vi "OuputFormater.vi"(9 "Sine in":fxp<+/-,16,0>[](array[numeric])=[0.0, 0.0, 0.0, 0.0, 0.0, 0.0, 0.0, 0.0], 10 "Cosine in":fxp<+/-,16,0>[](array[numeric])=[0.0, 0.0, 0.0, 0.0, 0.0, 0.0, 0.0, 0.0]) -> (3 "test":i16[](array[numeric]))   [LabVIEW 2013]
doc: "Outputs input from channel 0 as I*cos(t)-Q*sin(t) on analog output 0"
uses:
  <vilib>/eio/EIONode/EIONode.xnode
  <vilib>/rvi/FXPMathLib/FxpInterpret/XNode/nifxpmath_Interpret.xnode
  <vilib>/rvi/eio/common/nirviEmuTemplateMethod_errors.vi
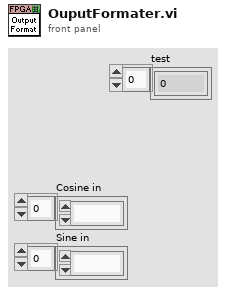
[diagram p1: front panel]
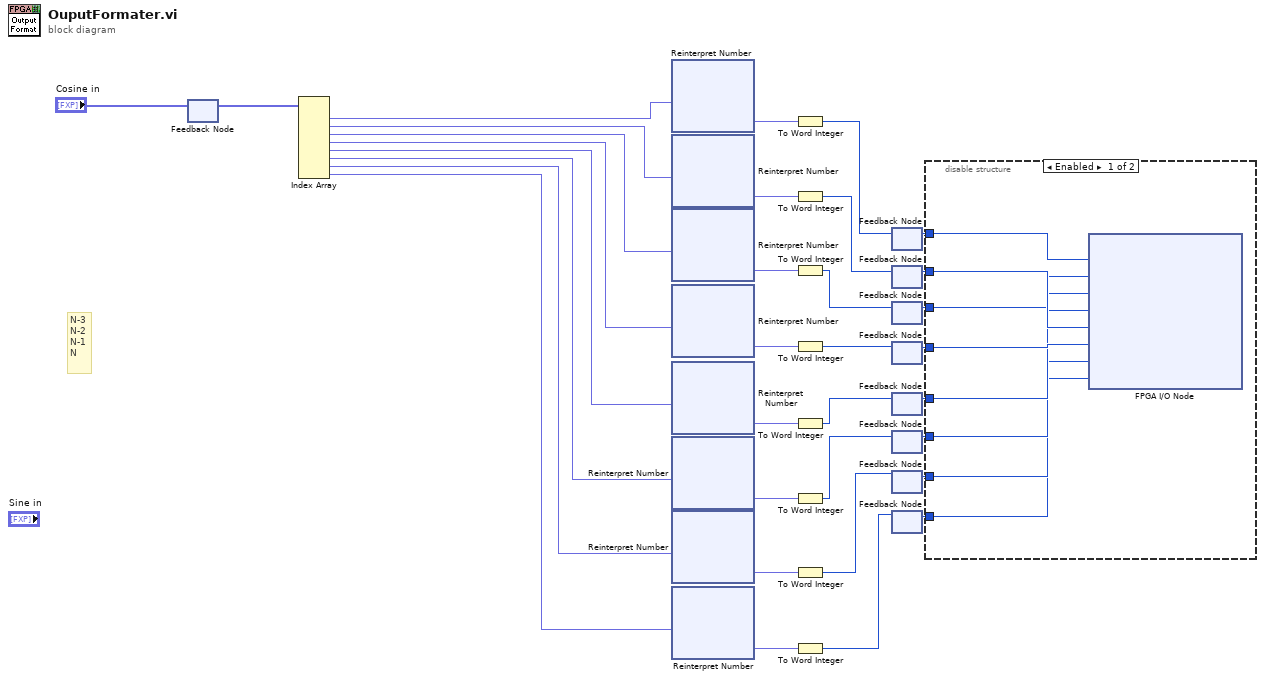
[diagram p0: block diagram]
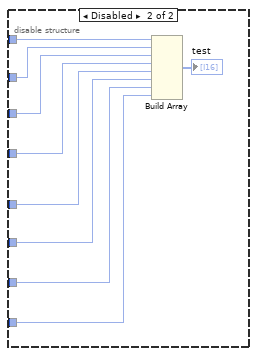
[diagram p2: hidden frame]
diagram:
  # "N-3\nN-2\nN-1\nN"
  n1 = feedback #1() -> (w34:fxp<+/-,16,0>[])  [unwired: 1 in]
  n2 = feedback-in #1("Cosine in") -> ()
  n3 = Index Array(array=w34) -> (element #1=w22:fxp<+/-,16,0>, element #2=w7:fxp<+/-,16,0>, element #3=w6:fxp<+/-,16,0>, element #4=w5:fxp<+/-,16,0>, element #5=w4:fxp<+/-,16,0>, element #6=w3:fxp<+/-,16,0>, element #7=w2:fxp<+/-,16,0>, element #8=w1:fxp<+/-,16,0>)  [unwired: 8 in]
  n4 = xnode "Reinterpret Number"("x"=w22) -> ("y"=w24:fxp<+/-,16,16>)
  n5 = xnode "Reinterpret Number"("x"=w7) -> ("y"=w21:fxp<+/-,16,16>)
  n6 = xnode "Reinterpret Number"("x"=w6) -> ("y"=w20:fxp<+/-,16,16>)
  n7 = xnode "Reinterpret Number"("x"=w5) -> ("y"=w19:fxp<+/-,16,16>)
  n8 = xnode "Reinterpret Number"("x"=w4) -> ("y"=w15:fxp<+/-,16,16>)
  n9 = xnode "Reinterpret Number"("x"=w3) -> ("y"=w16:fxp<+/-,16,16>)
  n10 = xnode "Reinterpret Number"("x"=w2) -> ("y"=w17:fxp<+/-,16,16>)
  n11 = xnode "Reinterpret Number"("x"=w1) -> ("y"=w18:fxp<+/-,16,16>)
  n12 = To Word Integer(number=w24) -> (16bit integer=w23:i16)
  n13 = To Word Integer(number=w21) -> (16bit integer=w14:i16)
  n14 = To Word Integer(number=w20) -> (16bit integer=w13:i16)
  n15 = To Word Integer(number=w19) -> (16bit integer=w12:i16)
  n16 = To Word Integer(number=w15) -> (16bit integer=w11:i16)
  n17 = To Word Integer(number=w16) -> (16bit integer=w10:i16)
  n18 = To Word Integer(number=w17) -> (16bit integer=w9:i16)
  n19 = To Word Integer(number=w18) -> (16bit integer=w8:i16)
  n20 = feedback #2() -> (w32:i16)  [unwired: 1 in]
  n21 = feedback-in #2(w23) -> ()
  n22 = feedback #3() -> (w31:i16)  [unwired: 1 in]
  n23 = feedback-in #3(w14) -> ()
  n24 = feedback #4() -> (w30:i16)  [unwired: 1 in]
  n25 = feedback-in #4(w13) -> ()
  n26 = feedback #5() -> (w29:i16)  [unwired: 1 in]
  n27 = feedback-in #5(w12) -> ()
  n28 = feedback #6() -> (w28:i16)  [unwired: 1 in]
  n29 = feedback-in #6(w11) -> ()
  n30 = feedback #7() -> (w27:i16)  [unwired: 1 in]
  n31 = feedback-in #7(w10) -> ()
  n32 = feedback #8() -> (w26:i16)  [unwired: 1 in]
  n33 = feedback-in #8(w9) -> ()
  n34 = feedback #9() -> (w25:i16)  [unwired: 1 in]
  n35 = feedback-in #9(w8) -> ()
  n36 = disable-structure shown="Enabled" {
    disable-tunnel: w32 -> [w42 w51]
    disable-tunnel: w31 -> [w41 w50]
    disable-tunnel: w30 -> [w40 w49]
    disable-tunnel: w29 -> [w39 w48]
    disable-tunnel: w28 -> [w38 w47]
    disable-tunnel: w27 -> [w37 w46]
    disable-tunnel: w26 -> [w36 w45]
    disable-tunnel: w25 -> [w35 w44]
    frame Enabled {
      n37 = xnode "FPGA I/O Node"("IO Module\\AO 0 N-3"=w42, "IO Module\\AO 0 N-2"=w40, "IO Module\\AO 0 N-1"=w38, "IO Module\\AO 0 N"=w36, "IO Module\\AO 1 N-3"=w41, "IO Module\\AO 1 N-2"=w39, "IO Module\\AO 1 N-1"=w37, "IO Module\\AO 1 N"=w35) -> ()  [unwired: 8 in, 8 out]
    }
    frame Disabled {
      n38 = Build Array(w51, w50, w49, w48, w47, w46, w45, w44) -> (→"test":i16[])
    }
  }
